vi "WfrmTest.vi"() -> ()   [LabVIEW 2014, in "WfrmPlugins.lvlib" / "C37Plugin.lvclass"]
uses:
  C37Plugin.lvclass
  <vilib>/imath/engines/lvmath2/RunTimeEngine/IndexRead/NIMS V(S).vi
  <instcachedir>/0/NIMS V(S)_0488751826AF41519A22953C041130DC.lvgen/NIMS V(S)_0488751826AF41519A22953C041130DC_000.vi
  <vilib>/imathl/engines/lvmath/Functions/Error Handling/Create Error.vi
  <vilib>/imath/engines/lvmath2/RunTimeEngine/RangeToken/NIMS_Range.vi
  <instcachedir>/0/NIMS_Range_9BCE657718DF4976A877346C61F22738.lvgen/NIMS_Range_9BCE657718DF4976A877346C61F22738_000.vi
  C:/Labview Data/MathScriptVIs/MCStatic_33564263232_7322b8936ace9060bcc211f5c44c036d.vi
  <instcachedir>/0/MCStatic_33564263232_7322b8936ace9060bcc211f5c44c036d_FD6C26AF7D604ED698836938523CBA8B.lvgen/MCStatic_33564263232_7322b8936ace9060bcc211f5c44c036d_FD6C26AF7D604ED698836938523CBA8B_000.vi
  <vilib>/imath/engines/lvmath2/RunTimeEngine/NodeEndStatement/NIMS_NodeEndStatement_Output.vi
  <instcachedir>/0/NIMS_NodeEndStatement_Output_53EC0D466D134D7ABD903AC30B43404B.lvgen/NIMS_NodeEndStatement_Output_53EC0D466D134D7ABD903AC30B43404B_005.vi
  <instcachedir>/0/NIMS_NodeEndStatement_Output_53EC0D466D134D7ABD903AC30B43404B.lvgen/NIMS_NodeEndStatement_Output_53EC0D466D134D7ABD903AC30B43404B_002.vi
  <vilib>/imath/engines/lvmath2/RunTimeEngine/ErrorHandling/NIMS_Finalize Error.vi
  Matlab/C37/genC37Signal.m
panel:
  in  "Settling":dbl=5.0
  out "time":dbl[](array[numeric])
  out "XY Graph":cluster{"Signal":dbl[], "time":dbl[]}(graph)
  in  "SignalParams":dbl[][](array[numeric])
  in  "End Time":dbl=5.0
  in  "Start Time":dbl
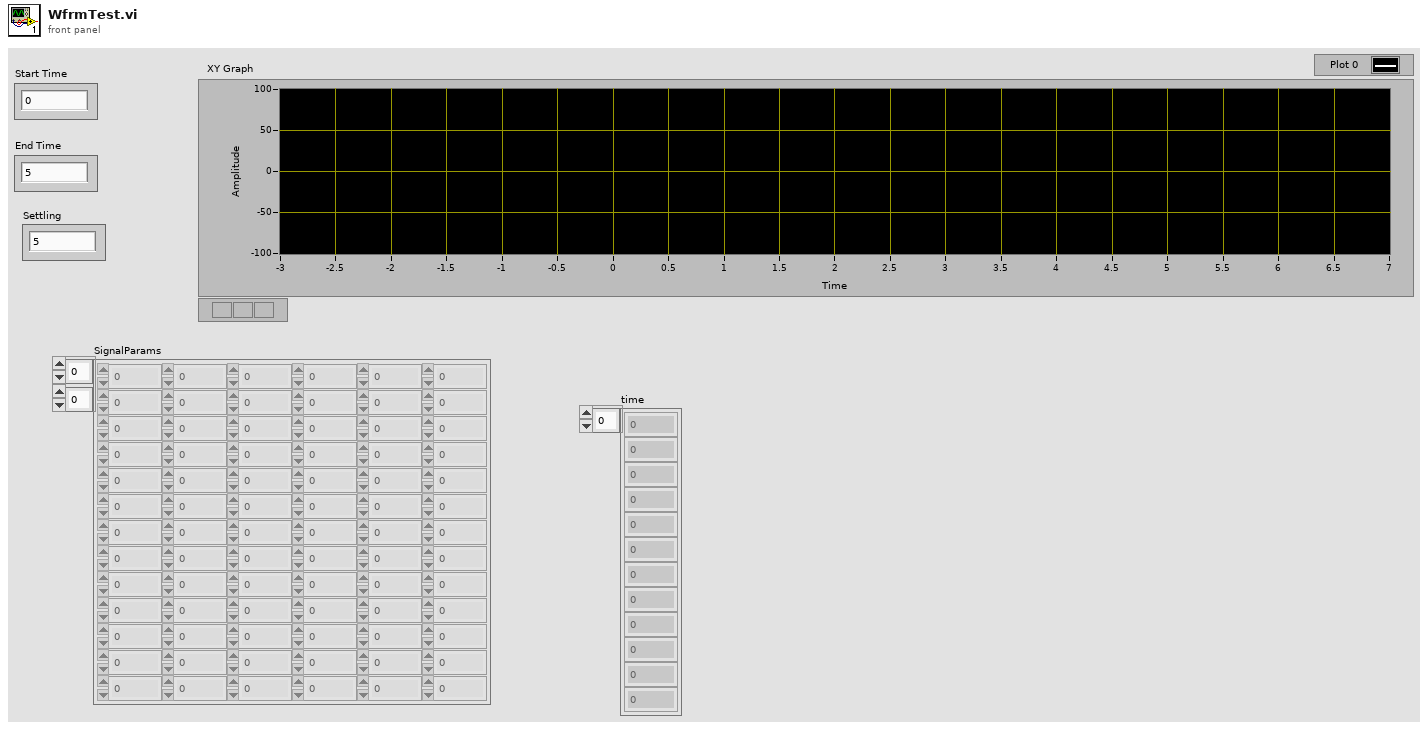
[diagram p1: front panel]
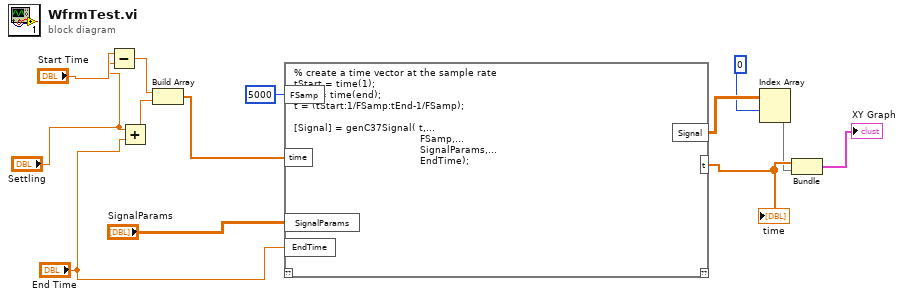
[diagram p0: block diagram]
diagram:
  n1 = Subtract(x="Start Time", y="Settling") -> (x-y=w4:dbl)
  n2 = Add(x="Settling", y="End Time") -> (x+y=w1:dbl)
  n3 = Build Array(w4, w1) -> (w6:dbl[])
  n4 = mathscript code="% create a time vector at the sample rate\ntStart = time(1);\ntEnd = time(end);\nt = (tStart:1/FSamp:tEnd-1/FSamp);\n\n[Signal] = genC37Signal( t,...\n                                          FSamp,...\n                                          SignalParams,...\n                                          EndTime);"("FSamp"=u32 5000, "time"=w6, "SignalParams"="SignalParams", "EndTime"="End Time") -> ("Signal"=w11:dbl[][], "t"=w8:dbl[])  [unwired: 1 in, 1 out]
  "time" <- w8
  n5 = Index Array(array=w11, index (row)=0) -> (element=w7:dbl[])  [unwired: 1 in]
  n6 = Bundle("t"=w8, "Signal"=w7) -> (→"XY Graph":cluster{"t":dbl[], "Signal":dbl[]})  [unwired: 1 in]
